vi "debug_camera_packages.vi"(8 "Detection Frame":T1 {"robots_blue"."height" format="%+4.3f"; "robots_blue"."pixel_y" format="%+4.3f"; "robots_blue"."pixel_x" format="%+4.3f"; "robots_blue"."orientation" format="%+4.3f"; "robots_blue"."y" format="%+4.3f"; "robots_blue"."confidence" format="%4.3f"; "robots_blue"."x" format="%+4.3f"; "robots_yellow"."height" format="%+4.3f"; "robots_yellow"."pixel_y" format="%+4.3f"; "robots_yellow"."pixel_x" format="%+4.3f"; "robots_yellow"."orientation" format="%+4.3f"; "robots_yellow"."y" format="%+4.3f"; "robots_yellow"."confidence" format="%4.3f"; "robots_yellow"."x" format="%+4.3f"}) -> ()   [LabVIEW 2017]
uses:
  SSL Detection Frame.ctl
  SSL Detection Robot.ctl
  <vilib>/Analysis/Matrix/Datatypes/RealMatrix.ctl
  SSL Detection Ball.ctl
  <vilib>/Analysis/Matrix/NI_Matrix.lvlib
panel:
  in  "file path (use dialog)":path
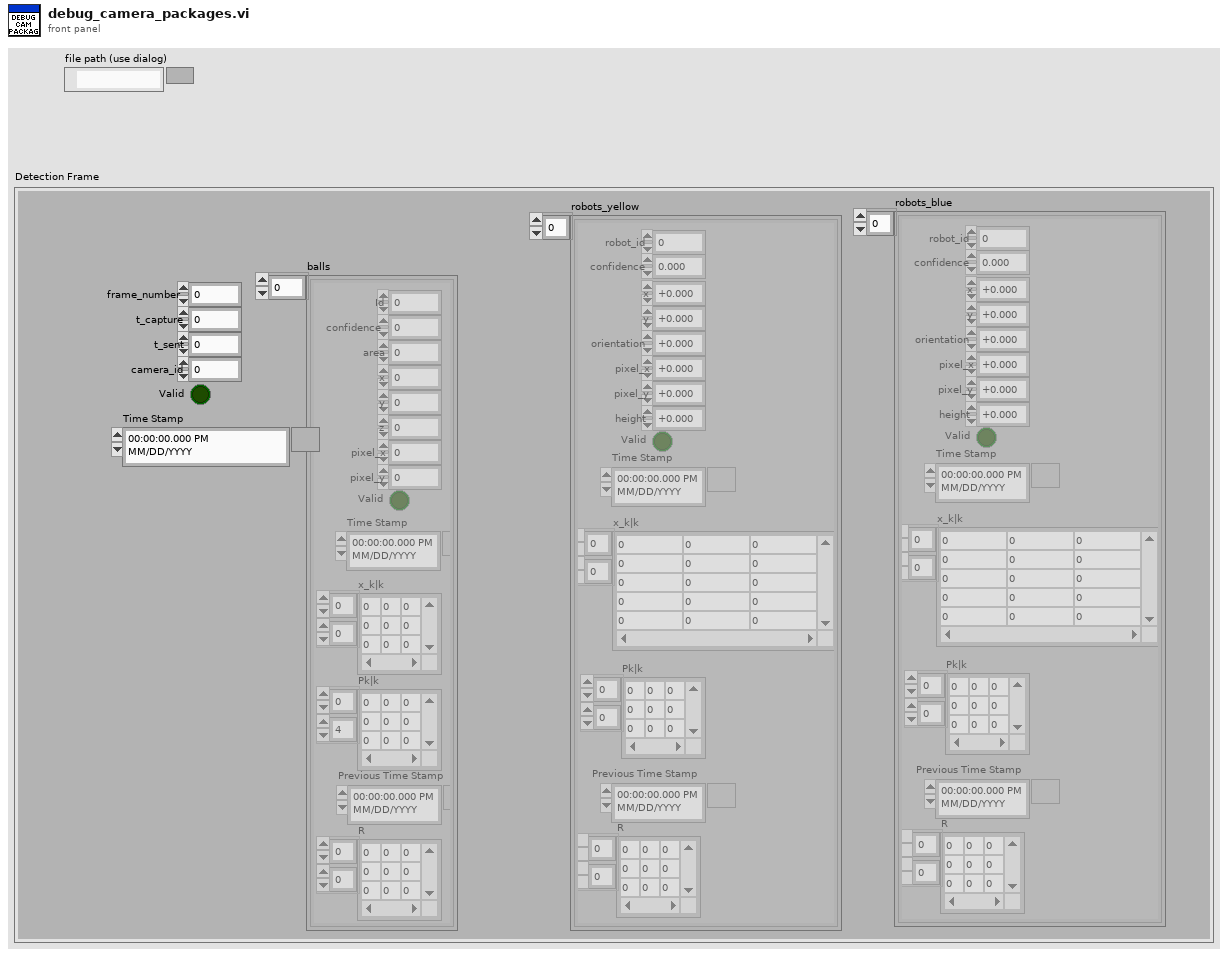
[diagram p1: front panel]
types:
  T1 = typedef "SSL Detection Frame.ctl" = cluster{"frame_number":u32, "t_capture":dbl, "t_sent":dbl, "camera_id":u32, "robots_yellow":T2[], "robots_blue":T2[], "balls":T4[], "Valid":bool, "Time Stamp":timestamp}
  T2 = typedef "SSL Detection Robot.ctl" = cluster{"x":sgl, "robot_id":u32, "confidence":sgl, "y":sgl, "orientation":sgl, "pixel_x":sgl, "pixel_y":sgl, "height":sgl, "Valid":bool, "Time Stamp":timestamp, "x_k|k":T3, "Pk|k":T3, "Previous Time Stamp":timestamp, "R":T3}
  T3 = typedef "NI_Matrix.lvlib/RealMatrix.ctl" = dbl[][]
  T4 = typedef "SSL Detection Ball.ctl" = cluster{"x":sgl, "area":u32, "confidence":sgl, "y":sgl, "z":sgl, "pixel_x":sgl, "pixel_y":sgl, "Valid":bool, "Time Stamp":timestamp, "x_k|k":T3, "Pk|k":T3, "Id":u32, "Previous Time Stamp":timestamp, "R":T3}
  T5 = enum16{"open", "replace", "create", "open or create", "replace or create", "replace or create with confirmation"}
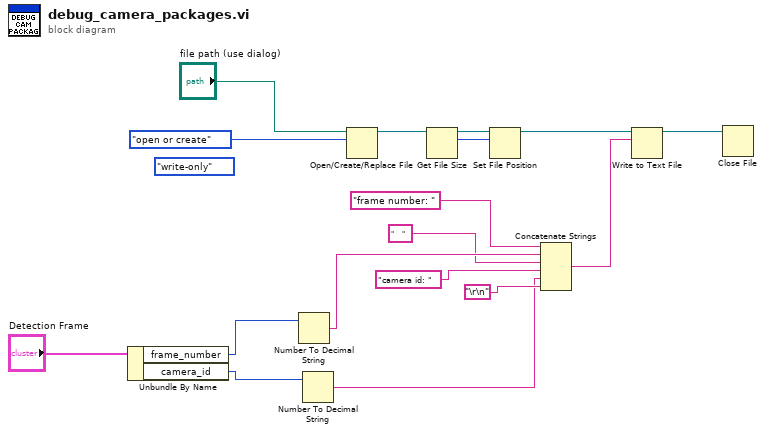
[diagram p0: block diagram]
diagram:
  (unwired) enum16{"read/write", "read-only", "write-only"}."write-only" ("access (0:read/write)")
  n1 = Unbundle By Name("Detection Frame") -> ("frame_number"=w7:u32, "camera_id"=w4:u32)
  n2 = Number To Decimal String(number=w7) -> (decimal integer string=w6:string)  [unwired: 1 in]
  n3 = Number To Decimal String(number=w4) -> (decimal integer string=w3:string)  [unwired: 1 in]
  n4 = Open/Create/Replace File(file path (use dialog)="file path (use dialog)", operation (0:open)=T5."open or create") -> (refnum out=w11:refnum<file>)  [unwired: 4 in, 2 out]
  n5 = Get File Size(file=w11) -> (refnum out=w9:refnum<file>, size (in bytes)=w10:i64)  [unwired: 1 in, 1 out]
  n6 = Set File Position(offset (in bytes) (0)=w10, refnum=w9) -> (refnum out=w2:refnum<file>)  [unwired: 2 in, 1 out]
  n7 = Concatenate Strings("frame number: " ("string"), w6, "    " ("string"), "camera id: " ("string"), w3, "\r\n") -> (w12:string)
  n8 = Write to Text File(file (use dialog)=w2, text=w12) -> (refnum out=w1:refnum<file>)  [unwired: 2 in, 2 out]
  n9 = Close File(refnum=w1) -> ()  [unwired: 1 in, 2 out]
